vi "TAT-Reporting.vi"(8 "error in (no error)":errorcluster) -> (0 "error out":errorcluster)   [LabVIEW 2017]
uses:
  <vilib>/addons/database/Connection.llb/DB Tools Open Connec (Path).vi
  <vilib>/Utility/file.llb/Write Delimited Spreadsheet (string).vi
  <vilib>/addons/database/NI_Database_API.lvlib
panel:
  in  "SELECT FILTER":string(combo)="PART_NO"
  in  "Export to Excel":bool
  out "DESCRIPTION":string
  out "Data History Table":string[][](table)
  in  "TO DATE":timestamp
  in  "FROM DATE":timestamp
  in  "Back":bool
  in  "Show Report":bool
  # "BARCODE VERIFICATION SYSTEM REPORTS"
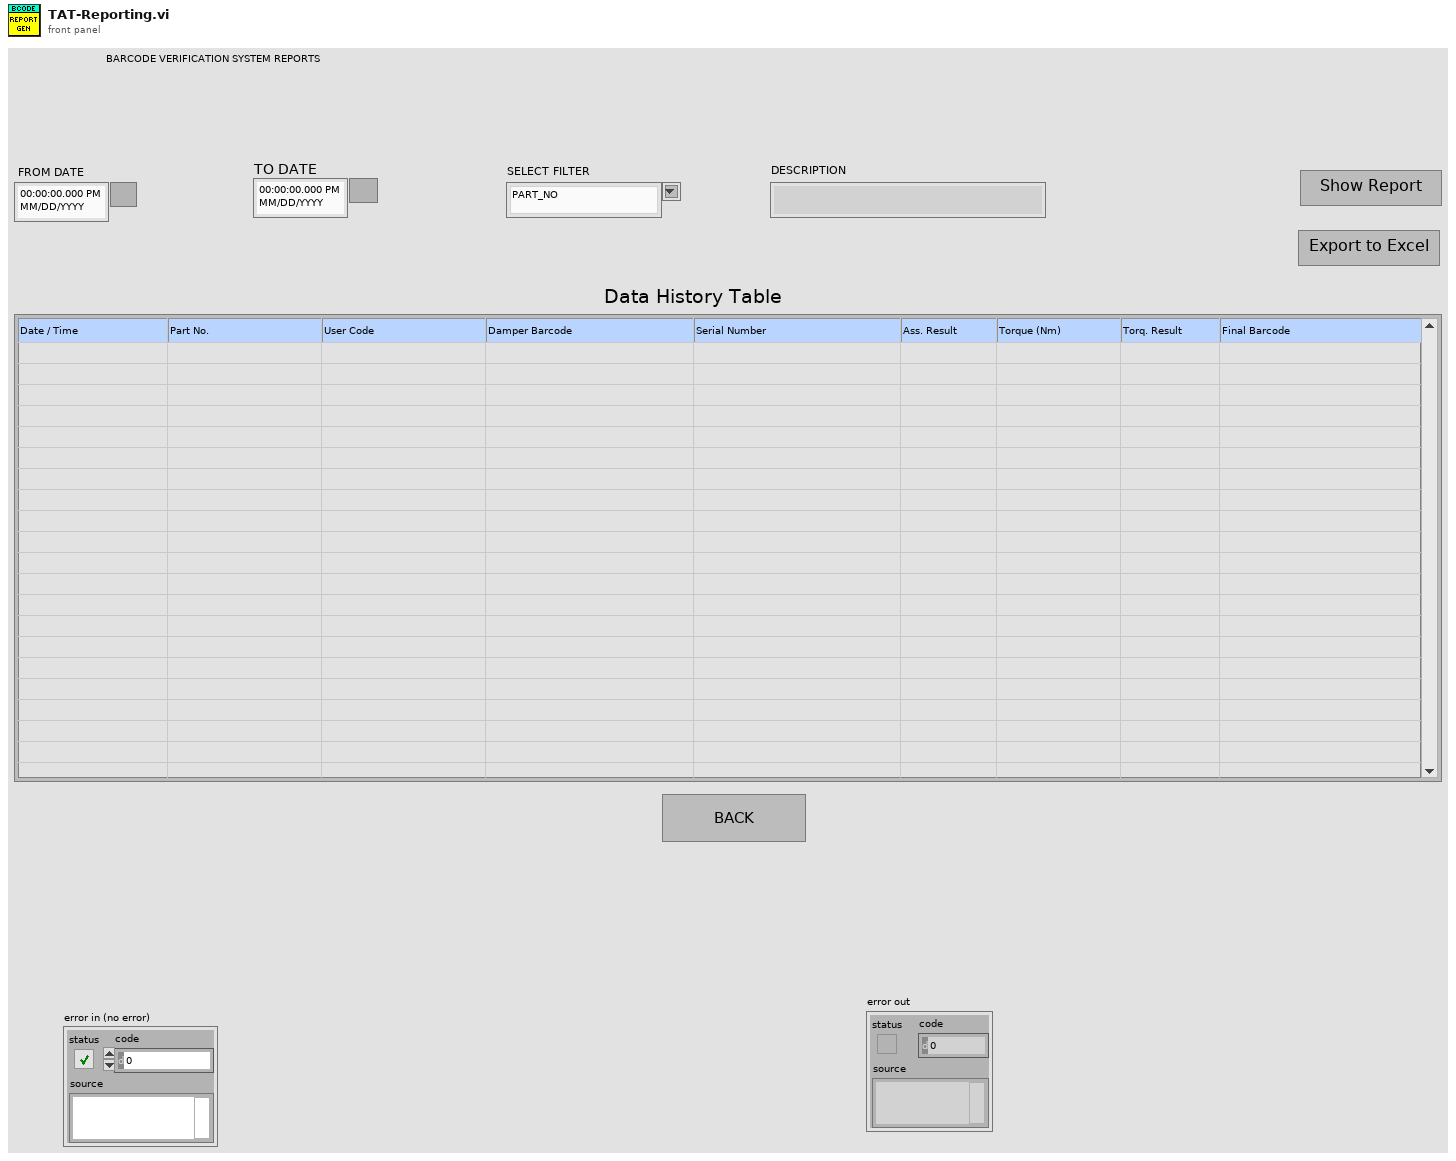
[diagram p1: front panel]
types:
  T1 = enum32{"invalid app kind", "Development System", "Run Time System", "Student Edition", "Embedded LabVIEW", "Evaluation", "Custom"}
  T2 = typedef "NI_Database_API.lvlib/Conn ObjectReference.ctl" = refnum<k1>
  T3 = typedef "LVRowAndColumnTypeDef.ctl" = cluster{"Row":i32, "Column":i32}
  T4 = enum32{"Invalid", "Standard", "Closed", "Hidden", "Minimized", "Maximized"}
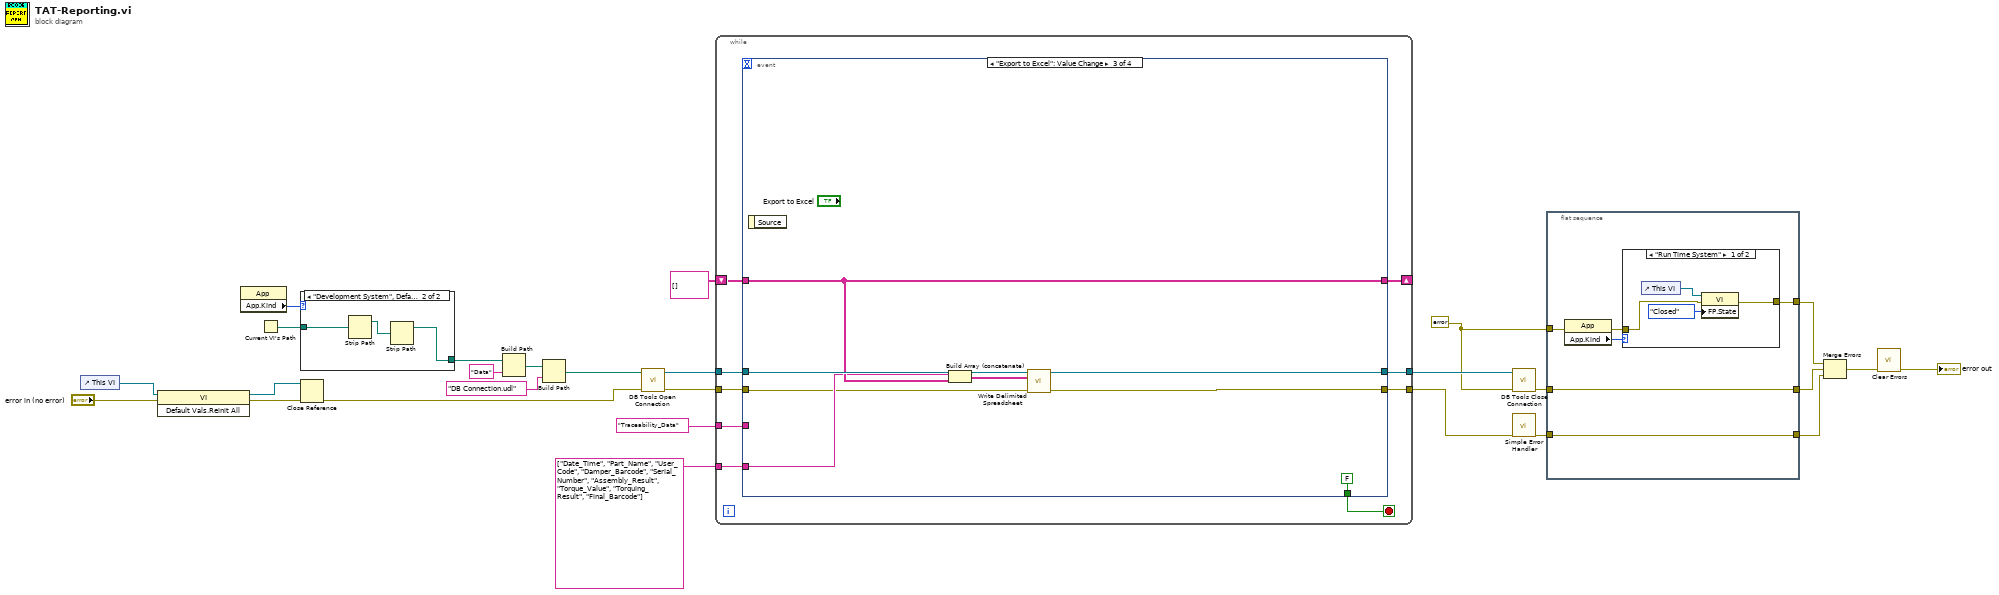
[diagram p0: block diagram]
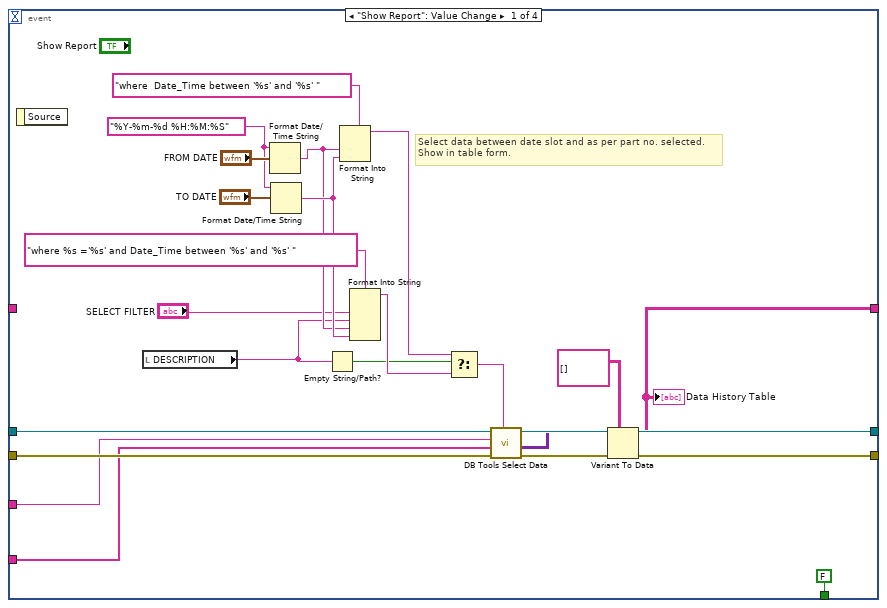
[diagram p3: hidden frame]
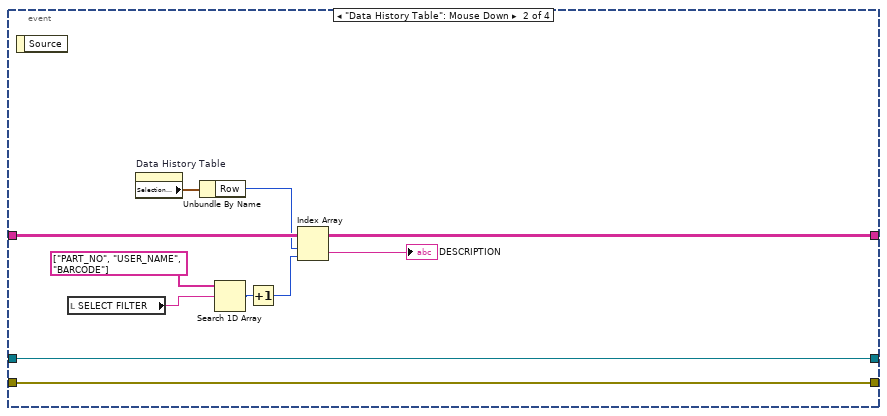
[diagram p4: hidden frame]
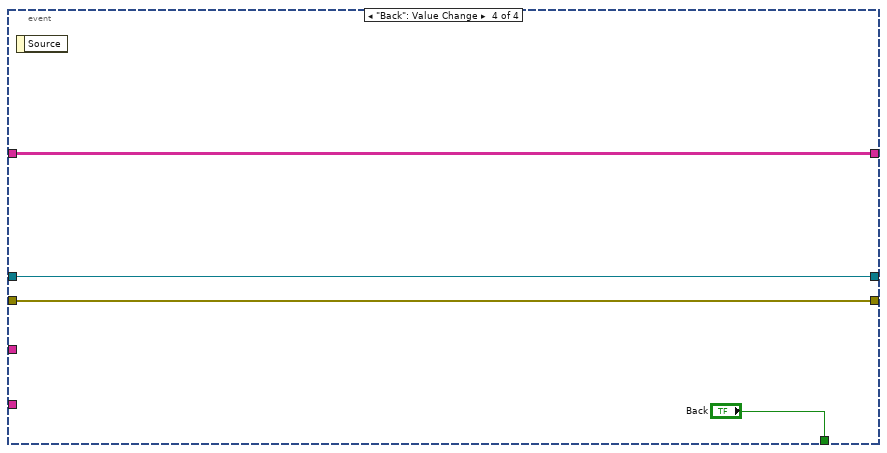
[diagram p5: hidden frame]
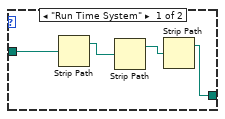
[diagram p6: hidden frame]
diagram:
  w13 = errorcluster {"status"=FALSE, "code"=0, "source"=""} ("error in (no error)")
  n1 = control-ref of="This VI"() -> (w7:refnum<vi>)
  n2 = invoke class="VI" method="Default Vals.Reinit All"(reference=w7, error in="error in (no error)") -> (reference out=w5:refnum<vi>, error out=w4:errorcluster)  [unwired: 1 in, 1 out]
  n3 = property class="App"() -> ("App.Kind"=w23:T1)  [unwired: 2 in, 2 out]
  n4 = Current VI's Path() -> (path=w24:path)
  n5 = case shown="\"Development System\", Default" w23 {
    tunnel: w24 -> [w29 w33]
    tunnel: [w28 w32] -> w21
    frame "Run Time System" {
      n6 = Strip Path(path=w29) -> (stripped path=w31:path)  [unwired: 1 out]
      n7 = Strip Path(path=w31) -> (stripped path=w30:path)  [unwired: 1 out]
      n8 = Strip Path(path=w30) -> (stripped path=w28:path)  [unwired: 1 out]
    }
    frame "Development System", Default {
      n9 = Strip Path(path=w33) -> (stripped path=w34:path)  [unwired: 1 out]
      n10 = Strip Path(path=w34) -> (stripped path=w32:path)  [unwired: 1 out]
    }
  }
  n11 = Close Reference(reference=w5, error in (no error)=w4) -> (error out=w3:errorcluster)
  n12 = Build Path(base path=w21, name or relative path="Data") -> (appended path=w22:path)
  n13 = Build Path(base path=w22, name or relative path="DB Connection.udl") -> (appended path=w18:path)
  n14 = call-poly <vilib>:"DB Tools Open Connection.vi"("error in (no error)"=w3, "connection information"=w18) -> ("error out"=w26:errorcluster, "connection reference"=w27:T2)  [unwired: 6 in]
  n15 = while {
    tunnel: string[] ["Date_Time", "Part_Name", "User_Code", "Damper_Barcode", "Serial_Number", "Assembly_Result", "Torque_Value", "Torquing_Result", "Final_Barcode"] -> [w39]
    tunnel: "Traceability_Data" ("table") -> [w38]
    tunnel: w27 -> [w43]
    tunnel: [w40] -> w25
    tunnel: w26 -> [w42]
    tunnel: [w41] -> w16
    shift-right: [w36] -> _
    shift-left: string[][] [] -> [w35]
    stop <- w37 stop-if-true
    n16 = event shown="[2] \"Export to Excel\": Value Change" {
      selector: _ -> [_ _ _ _]
      dyn-events: _ -> [_ _ _ _]
      timeout: _ -> [_ _ _ _]
      tunnel: w43 -> [w67 w74 w84 w87]
      tunnel: w42 -> [w66 w73 w79 w86]
      tunnel: [w58 w73 w78 w86] -> w41
      tunnel: [w65 w74 w84 w87] -> w40
      tunnel: w39 -> [w64 _ w80 _]
      tunnel: w38 -> [w63 _ _ _]
      tunnel: [FALSE ("Back") _ FALSE ("Back") "Back"] -> w37
      tunnel: [w48 w77 w81 w85] -> w36
      tunnel: w35 -> [_ w77 w81 w85]
      event "Show Report": Value Change {
        w51 = "%Y-%m-%d %H:%M:%S"
        # "Select data between date slot and as per part no. selected.\nShow in table form."
        n17 = event-data() -> ()  [unwired: 1 in, 1 out]
        n18 = local read "DESCRIPTION"() -> (w44:string)
        n19 = Format Date/Time String(time format string (%c)=w51, seconds (now)="FROM DATE") -> (date/time string=w46:string)  [unwired: 1 in]
        n20 = Format Date/Time String(time format string (%c)=w51, seconds (now)="TO DATE") -> (date/time string=w47:string)  [unwired: 1 in]
        n21 = Empty String/Path?(string/path=w44) -> (empty?=w49:bool)
        n22 = Format Into String(format string="where  Date_Time between '%s' and '%s' ", w46, w47) -> (resulting string=w56:string)  [unwired: 2 in, 1 out]
        n23 = Format Into String(format string="where %s ='%s' and Date_Time between '%s' and '%s' ", "SELECT FILTER", w44, w46, w47) -> (resulting string=w57:string)  [unwired: 2 in, 1 out]
        n24 = Select(t=w56, s=w49, f=w57) -> (s? t:f=w50:string)
        n25 = call <vilib>:"DB Tools Select Data.vi"("condition"=w50, "error in (no error)"=w66, "columns"=w64, "table"=w63, "connection reference"=w67) -> ("error out"=w59:errorcluster, "data"=w62:variant[][], "connection reference out"=w65:T2)  [unwired: 1 in]
        n26 = Variant To Data(error in=w59, type=string[][] [], Variant=w62) -> (data=w48:string[][], error out=w58:errorcluster)
        "Data History Table" <- w48
      }
      event "Data History Table": Mouse Down {
        n27 = event-data() -> ()  [unwired: 1 in, 1 out]
        n28 = local read "SELECT FILTER"() -> (w70:string)
        n29 = property on="Data History Table" class="Tbl (strict)"() -> ("Selection Start"=w76:T3)  [unwired: 2 in, 2 out]
        n30 = Unbundle By Name(w76) -> ("Row"=w75:i32)
        n31 = Search 1D Array(1D array=string[] ["PART_NO", "USER_NAME", "BARCODE"], element=w70) -> (index of element=w69:i32)  [unwired: 1 in]
        n32 = Increment(x=w69) -> (x+1=w68:i32)
        n33 = Index Array(array=w77, index (row)=w75, index (col)=w68) -> (element=→"DESCRIPTION":string)
      }
      event "Export to Excel": Value Change {
        n34 = event-data() -> ()  [unwired: 1 in, 1 out]
        n35 = Build Array (concatenate)(w80, w81) -> (w82:string[][])
        n36 = call-poly <vilib>:"Write Delimited Spreadsheet.vi"("2D data"=w82, "error in (no error)"=w79) -> ("error out"=w78:errorcluster)  [unwired: 12 in, 1 out]
      }
      event "Back": Value Change {
        n37 = event-data() -> ()  [unwired: 1 in, 1 out]
      }
    }
  }
  n38 = call <vilib>:"DB Tools Close Connection.vi"("error in (no error)"=w13, "connection reference"=w25) -> ("error out"=w11:errorcluster)  [unwired: 5 in]
  n39 = call <vilib>:"Simple Error Handler.vi"("error in (no error)"=w16) -> ("error out"=w9:errorcluster)  [unwired: 4 in, 4 out]
  n40 = flat-sequence {
    tunnel: [w92] -> w14
    tunnel: w13 -> [w91]
    tunnel: [w90] -> w12
    tunnel: w11 -> [w90]
    tunnel: [w89] -> w10
    tunnel: w9 -> [w89]
    frame #0 {
      n41 = property class="App"(error in=w91) -> (error out=w93:errorcluster, "App.Kind"=w94:T1)  [unwired: 1 in, 1 out]
      n42 = case shown="\"Run Time System\"" w94 {
        tunnel: w93 -> [w96 w99]
        tunnel: [w95 w99] -> w92
        frame "Run Time System" {
          n43 = control-ref of="This VI"() -> (w98:refnum<vi>)
          n44 = property class="VI"(reference=w98, error in=w96, "FP.State"=T4."Closed" ("Front Panel Window:State")) -> (error out=w95:errorcluster)  [unwired: 1 out]
        }
        frame "Development System", Default {
        }
      }
    }
  }
  n45 = Merge Errors(w14, w12, w10) -> (w15:errorcluster)
  n46 = call <vilib>:"Clear Errors.vi"("error in (no error)"=w15) -> ("error out"=→"error out":errorcluster)  [unwired: 5 in, 1 out]
